vi "main2.vi"() -> ()   [LabVIEW 2016]
uses:
  <vilib>/platform/TimedLoop/XDataNode/XDataNode.xnode
  <vilib>/Platform/TimedLoop/XDataNode/nitl_modes.ctl
  <vilib>/Platform/TimedLoop/XDataNode/XDNodeRunTimeDep.lvlib
  <vilib>/Platform/TimedLoop/XDataNode/wakeup.ctl
  <vilib>/Platform/TimedLoop/XDataNode/timing_clust.ctl
panel:
  in  "retake readings":bool
  in  "Multimeter\nMeasurement":u16(ring) caption="Measurement" items=["DC Voltage (50 A - 50 mV Shunt)", "DC Current (3 A Terminal)", "DC Current (10 A Terminal)", "AC Voltage (50 A - 50 mV Shunt)", "AC Current (3 A Terminal)", "AC Current (10 A Terminal)", "DC Voltage (other)", "AC Voltage (other)", "Continuity", "Diode", "Frequency", "Resistance 4-wire", "Period", "Resistance 2-wire", "Temperature", "DC Voltage Ratio", "Capacitance"]
  in  "zero Hall sensor 3":bool
  in  "zero Hall sensor 2":bool
  in  "zero Hall sensor 1":bool
  in  "start measurement":bool
  in  "initalize instuments":bool
  in  "take readings":bool
  in  "stop":bool
  in  "duration":dbl format="%<%H:%M:%S>t"
  in  "number of readings":i32
  in  "temperature monitor.on":bool
  in  "multimeter.on":bool
  in  "gaussmeter 3.on":bool
  in  "gaussmeter 2.on":bool
  in  "gaussmeter 1.on":bool
  out "status temperature monitor":bool
  out "status multimeter":bool
  out "status gaussmeter 3":bool
  out "status gaussmeter 2":bool
  out "status gaussmeter 1":bool
  in  "VISA resource name temperature monitor":refnum<visa-resource-name>
  in  "VISA resource name multimeter":refnum<visa-resource-name>
  in  "VISA resource name gaussmeter 3":refnum<visa-resource-name>
  in  "VISA resource name gaussmeter 2":refnum<visa-resource-name>
  in  "VISA resource name gaussmeter 1":refnum<visa-resource-name>
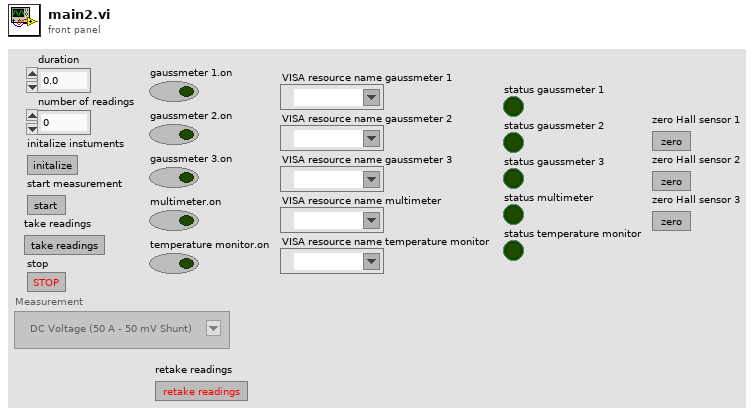
[diagram p1: front panel]
types:
  T1 = enum8{"Enabled", "Disabled", "Disabled and Grayed Out"}
  T2 = typedef "XDNodeRunTimeDep.lvlib/timing_clust.ctl" = cluster{"Expected End [f-1]":u64, "Actual End [f-1]":u64, "Finished Late? [f-1]":bool, "Expected End [i-1]":u64, "Actual End [i-1]":u64, "Finished Late? [i-1]":bool, "Expected Start [i]":u64, "Actual Start [i]":u64, "Expected Start [f]":u64, "Actual Start [f]":u64, "Source Name":string, "Structure Name":string, "Period":i64, "Deadline":i64, "Offset":i64, "Start":i64, "Priority":i32, "Timeout":i32, "Mode":T3, "Wakeup Reason":T4, "Error":errorcluster, "Source Type":string, "Secondary Source Type":string, "Global End Time":u64, "Global Start Time":u64, "Frame Duration":u64, "Iteration Duration":u64, "Assigned CPU":i32, "I/O Scan Engine Mode":u32}
  T3 = typedef "XDNodeRunTimeDep.lvlib/nitl_modes.ctl" = enum32{"No Change", "Process missed periods, maintain original phase", "Discard missed periods, maintain original phase", "Process missed periods, ignore original phase", "Discard missed periods, ignore original phase"}
  T4 = typedef "XDNodeRunTimeDep.lvlib/wakeup.ctl" = enum32{"Normal", "Aborted", "Asynchronous wakeup", "Timing source error", "Timed loop error", "Timeout"}
  T5 = cluster{"gaussmeter 1":cluster{"VISA recourse name":refnum<visa-resource-name>, "on":bool, "header text":string, "units":i32, "initalization successfull":bool}, "gaussmeter 2":cluster{"VISA recourse name":refnum<visa-resource-name>, "on":bool, "header text":string, "units":i32, "initalization successfull":bool}, "gaussmeter 3":cluster{"VISA recourse name":refnum<visa-resource-name>, "on":bool, "header text":string, "units":i32, "initalization successfull":bool}, "multimeter":cluster{"VISA recourse name":refnum<visa-resource-name>, "on":bool, "header text":string, "units":i32, "initalization successfull":bool}, "temperature monitor":cluster{"VISA recourse name":refnum<visa-resource-name>, "on":bool, "header text":string, "units":i32, "initalization successfull":bool}, "duration":cluster{"not zero":bool, "duration":dbl, "start time":dbl}}
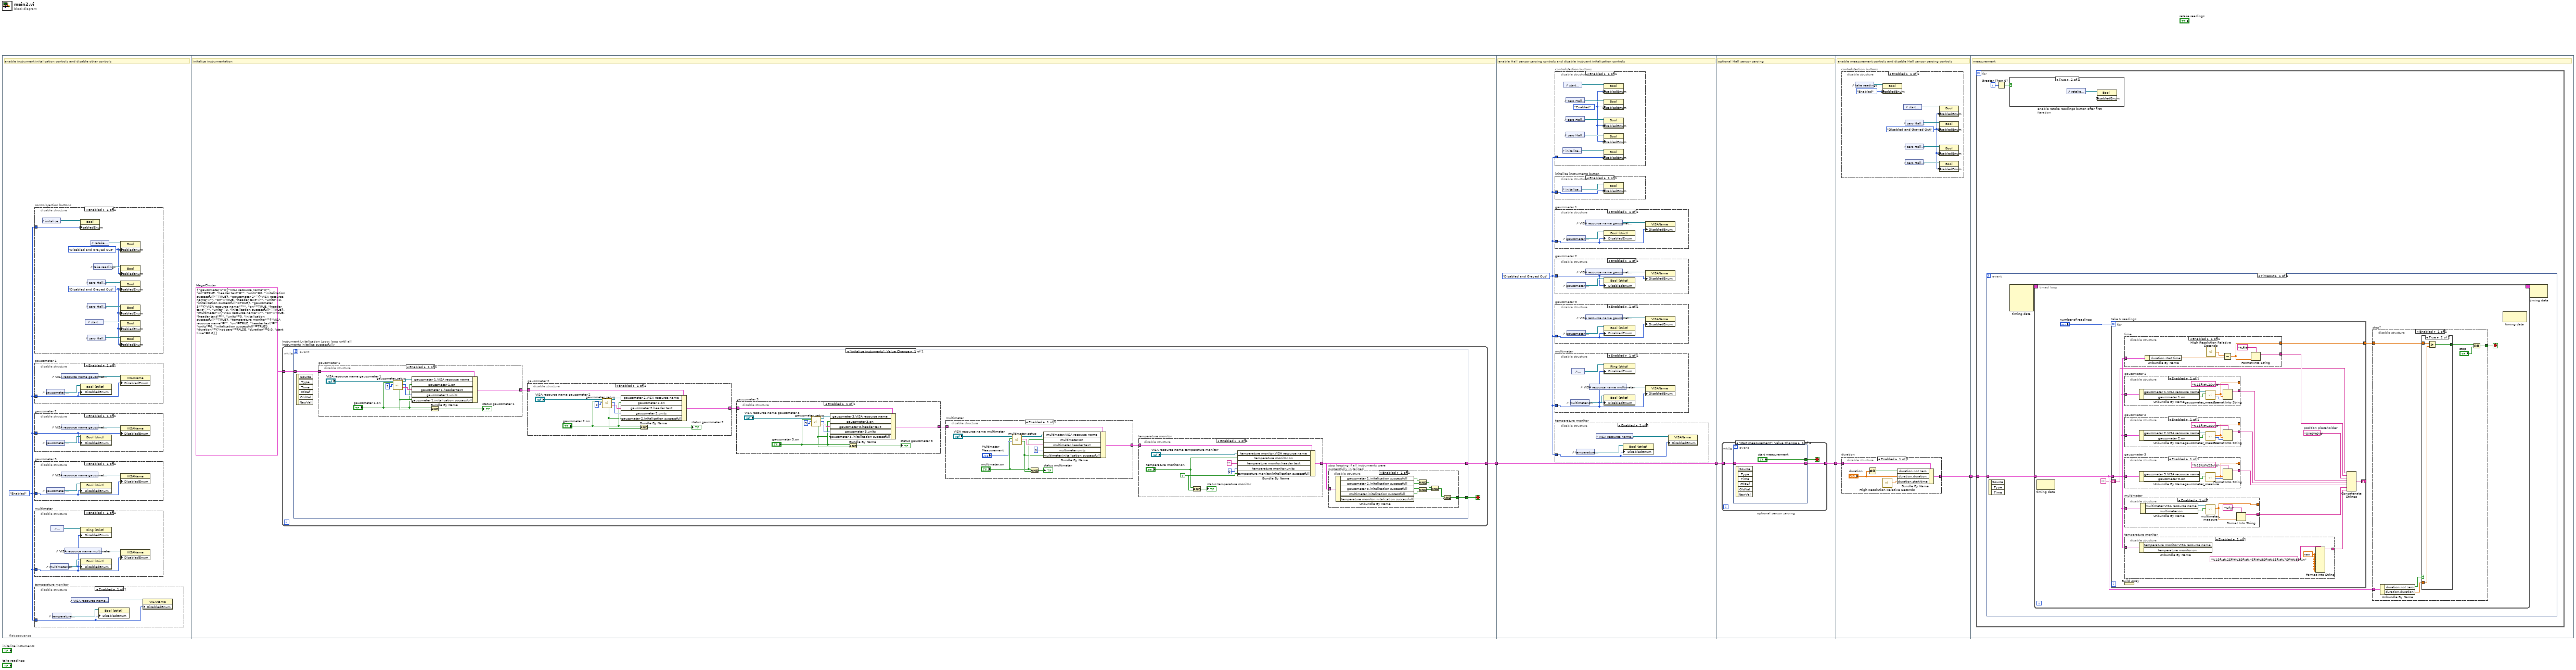
[diagram p0: block diagram]
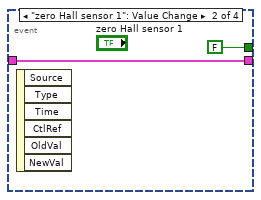
[diagram p2: hidden frame]
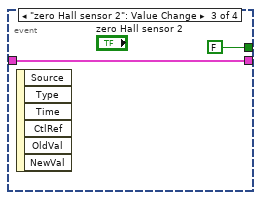
[diagram p3: hidden frame]
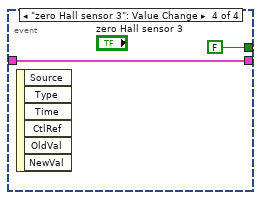
[diagram p4: hidden frame]
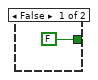
[diagram p6: hidden frame]
diagram:
  n1 = flat-sequence {
    tunnel: [w33] -> w2
    tunnel: w2 -> [w103]
    tunnel: [w103] -> w1
    tunnel: [w130] -> w3
    tunnel: w1 -> [w129]
    tunnel: [w143] -> w4
    tunnel: w3 -> [w142]
    tunnel: w4 -> [w156]
    frame #0 {
      w5 = T1."Enabled" ("Disabled")
      # "enable instrument initalization controls and disable other controls"
      n2 = disable-structure "controls/action buttons" shown="Enabled" {
        disable-tunnel: w5 -> [w12]
        frame Enabled {
          w6 = T1."Disabled and Grayed Out" ("Disabled")
          w8 = T1."Disabled and Grayed Out" ("Disabled")
          n3 = control-ref of="initalize instuments"() -> (w13:refnum<vi>)
          n4 = property class="Bool"(reference=w13, "DisabledEnum"=w12) -> ()  [unwired: 1 in, 2 out]
          n5 = control-ref of="start measurement"() -> (w15:refnum<vi>)
          n6 = control-ref of="zero Hall sensor 2"() -> (w10:refnum<vi>)
          n7 = control-ref of="zero Hall sensor 1"() -> (w11:refnum<vi>)
          n8 = control-ref of="zero Hall sensor 3"() -> (w9:refnum<vi>)
          n9 = control-ref of="retake readings"() -> (w7:refnum<vi>)
          n10 = control-ref of="take readings"() -> (w14:refnum<vi>)
          n11 = property class="Bool"(reference=w7, "DisabledEnum"=w6) -> ()  [unwired: 1 in, 2 out]
          n12 = property class="Bool"(reference=w14, "DisabledEnum"=w6) -> ()  [unwired: 1 in, 2 out]
          n13 = property class="Bool"(reference=w10, "DisabledEnum"=w8) -> ()  [unwired: 1 in, 2 out]
          n14 = property class="Bool"(reference=w11, "DisabledEnum"=w8) -> ()  [unwired: 1 in, 2 out]
          n15 = property class="Bool"(reference=w15, "DisabledEnum"=w8) -> ()  [unwired: 1 in, 2 out]
          n16 = property class="Bool"(reference=w9, "DisabledEnum"=w8) -> ()  [unwired: 1 in, 2 out]
        }
      }
      n17 = disable-structure "gaussmeter 1" shown="Enabled" {
        disable-tunnel: w5 -> [w29]
        frame Enabled {
          n18 = control-ref of="gaussmeter 1.on"() -> (w30:refnum<vi>)
          n19 = control-ref of="VISA resource name gaussmeter 1"() -> (w31:refnum<vi>)
          n20 = property class="Bool (strict)"(reference=w30, "DisabledEnum"=w29) -> ()  [unwired: 1 in, 2 out]
          n21 = property class="VISAName"(reference=w31, "DisabledEnum"=w29) -> ()  [unwired: 1 in, 2 out]
        }
      }
      n22 = disable-structure "gaussmeter 2" shown="Enabled" {
        disable-tunnel: w5 -> [w26]
        frame Enabled {
          n23 = control-ref of="gaussmeter 2.on"() -> (w27:refnum<vi>)
          n24 = control-ref of="VISA resource name gaussmeter 2"() -> (w28:refnum<vi>)
          n25 = property class="Bool (strict)"(reference=w27, "DisabledEnum"=w26) -> ()  [unwired: 1 in, 2 out]
          n26 = property class="VISAName"(reference=w28, "DisabledEnum"=w26) -> ()  [unwired: 1 in, 2 out]
        }
      }
      n27 = disable-structure "gaussmeter 3" shown="Enabled" {
        disable-tunnel: w5 -> [w16]
        frame Enabled {
          n28 = control-ref of="gaussmeter 3.on"() -> (w17:refnum<vi>)
          n29 = control-ref of="VISA resource name gaussmeter 3"() -> (w18:refnum<vi>)
          n30 = property class="Bool (strict)"(reference=w17, "DisabledEnum"=w16) -> ()  [unwired: 1 in, 2 out]
          n31 = property class="VISAName"(reference=w18, "DisabledEnum"=w16) -> ()  [unwired: 1 in, 2 out]
        }
      }
      n32 = disable-structure "multimeter" shown="Enabled" {
        disable-tunnel: w5 -> [w22]
        frame Enabled {
          n33 = control-ref of="multimeter.on"() -> (w24:refnum<vi>)
          n34 = control-ref of="Multimeter\nMeasurement"() -> (w25:refnum<vi>)
          n35 = control-ref of="VISA resource name multimeter"() -> (w23:refnum<vi>)
          n36 = property class="Ring (strict)"(reference=w25, "DisabledEnum"=w22) -> ()  [unwired: 1 in, 2 out]
          n37 = property class="Bool (strict)"(reference=w24, "DisabledEnum"=w22) -> ()  [unwired: 1 in, 2 out]
          n38 = property class="VISAName"(reference=w23, "DisabledEnum"=w22) -> ()  [unwired: 1 in, 2 out]
        }
      }
      n39 = disable-structure "temperature monitor" shown="Enabled" {
        disable-tunnel: w5 -> [w21]
        frame Enabled {
          n40 = control-ref of="temperature monitor.on"() -> (w19:refnum<vi>)
          n41 = control-ref of="VISA resource name temperature monitor"() -> (w20:refnum<vi>)
          n42 = property class="Bool (strict)"(reference=w19, "DisabledEnum"=w21) -> ()  [unwired: 1 in, 2 out]
          n43 = property class="VISAName"(reference=w20, "DisabledEnum"=w21) -> ()  [unwired: 1 in, 2 out]
        }
      }
    }
    frame #1 {
      w32 = T5 {"gaussmeter 1"={"VISA recourse name"="", "on"=TRUE, "header text"="", "units"=0, "initalization successfull"=TRUE}, "gaussmeter 2"={"VISA recourse name"="", "on"=TRUE, "header text"="", "units"=0, "initalization successfull"=TRUE}, "gaussmeter 3"={"VISA recourse name"="", "on"=TRUE, "header text"="", "units"=0, "initalization successfull"=TRUE}, "multimeter"={"VISA recourse name"="", "on"=TRUE, "header text"="", "units"=0, "initalization successfull"=TRUE}, "temperature monitor"={"VISA recourse name"="", "on"=TRUE, "header text"="", "units"=0, "initalization successfull"=TRUE}, "duration"={"not zero"=FALSE, "duration"=0.0, "start time"=0.0}}  # MegaCluster
      # "initalize instrumentation"
      n44 = while "Instrument Lnitalization Loop: loop until all instruments initalize successfully" {
        tunnel: [w35] -> w33
        tunnel: w32 -> [w36]
        stop <- w34 stop-if-true
        n45 = event shown="[0] \"initalize instuments\": Value Change" {
          selector: _ -> [_]
          dyn-events: _ -> [_]
          timeout: _ -> [_]
          tunnel: w36 -> [w39]
          tunnel: [w38] -> w35
          tunnel: [w37] -> w34
          event "initalize instuments": Value Change {
            n46 = event-data() -> ()  [unwired: 1 in, 6 out]
            n47 = disable-structure "gaussmeter 1" shown="Enabled" {
              disable-tunnel: [w81] -> w43
              disable-tunnel: w39 -> [w80]
              frame Enabled {
                n48 = call "gaussmeter_setup.vi"("VISA resource name Gaussmeter"="VISA resource name gaussmeter 1", "Switch Gaussmeter"="gaussmeter 1.on", "Gaussmeter Number"=u8 1) -> ("Status Gaussmeter"=w73:bool, "Gaussmeter VISA resource name out"=w77:refnum<visa-resource-name>, "Field Units"=w75:u16, "Text Output"=w76:string)  [unwired: 6 in, 7 out]
                n49 = Bundle By Name(cluster=w80, "gaussmeter 1.VISA recourse name"=w77, "gaussmeter 1.on"="gaussmeter 1.on", "gaussmeter 1.header text"=w76, "gaussmeter 1.units"=w75, "gaussmeter 1.initalization successfull"=w73) -> (w81:T5)
                n50 = And(x="gaussmeter 1.on", y=w73) -> (x .and. y?=→"status gaussmeter 1":bool)
              }
            }
            n51 = disable-structure "gaussmeter 2" shown="Enabled" {
              disable-tunnel: [w100] -> w42
              disable-tunnel: w43 -> [w101]
              frame Enabled {
                n52 = call "gaussmeter_setup.vi"("VISA resource name Gaussmeter"="VISA resource name gaussmeter 2", "Switch Gaussmeter"="gaussmeter 2.on", "Gaussmeter Number"=u8 2) -> ("Status Gaussmeter"=w93:bool, "Gaussmeter VISA resource name out"=w97:refnum<visa-resource-name>, "Field Units"=w96:u16, "Text Output"=w95:string)  [unwired: 6 in, 7 out]
                n53 = Bundle By Name(cluster=w101, "gaussmeter 2.VISA recourse name"=w97, "gaussmeter 2.on"="gaussmeter 2.on", "gaussmeter 2.header text"=w95, "gaussmeter 2.units"=w96, "gaussmeter 2.initalization successfull"=w93) -> (w100:T5)
                n54 = And(x="gaussmeter 2.on", y=w93) -> (x .and. y?=→"status gaussmeter 2":bool)
              }
            }
            n55 = disable-structure "gaussmeter 3" shown="Enabled" {
              disable-tunnel: [w91] -> w41
              disable-tunnel: w42 -> [w90]
              frame Enabled {
                n56 = call "gaussmeter_setup.vi"("VISA resource name Gaussmeter"="VISA resource name gaussmeter 3", "Switch Gaussmeter"="gaussmeter 3.on", "Gaussmeter Number"=u8 3) -> ("Status Gaussmeter"=w82:bool, "Gaussmeter VISA resource name out"=w88:refnum<visa-resource-name>, "Field Units"=w85:u16, "Text Output"=w86:string)  [unwired: 6 in, 7 out]
                n57 = Bundle By Name(cluster=w90, "gaussmeter 3.VISA recourse name"=w88, "gaussmeter 3.on"="gaussmeter 3.on", "gaussmeter 3.header text"=w86, "gaussmeter 3.units"=w85, "gaussmeter 3.initalization successfull"=w82) -> (w91:T5)
                n58 = And(x="gaussmeter 3.on", y=w82) -> (x .and. y?=→"status gaussmeter 3":bool)
              }
            }
            n59 = disable-structure "multimeter" shown="Enabled" {
              disable-tunnel: [w71] -> w40
              disable-tunnel: w41 -> [w70]
              frame Enabled {
                n60 = call "multimeter_setup.vi"("Measurement"="Multimeter\nMeasurement", "Switch"="multimeter.on", "VISA resource name"="VISA resource name multimeter") -> ("status"=w62:bool, "text"=w66:string, "VISA resource name out"=w67:refnum<visa-resource-name>)  [unwired: 5 in, 1 out]
                n61 = And(x="multimeter.on", y=w62) -> (x .and. y?=→"status multimeter":bool)
                n62 = Bundle By Name(cluster=w70, "multimeter.VISA recourse name"=w67, "multimeter.on"="multimeter.on", "multimeter.header text"=w66, "multimeter.units"=0, "multimeter.initalization successfull"=w62) -> (w71:T5)
              }
            }
            n63 = disable-structure "temperature monitor" shown="Enabled" {
              disable-tunnel: [w61] -> w38
              disable-tunnel: w40 -> [w60]
              frame Enabled {
                w55 = TRUE
                n64 = And(x="temperature monitor.on", y=w55) -> (x .and. y?=→"status temperature monitor":bool)
                n65 = Bundle By Name(cluster=w60, "temperature monitor.VISA recourse name"="VISA resource name temperature monitor", "temperature monitor.on"="temperature monitor.on", "temperature monitor.header text"="", "temperature monitor.units"=0, "temperature monitor.initalization successfull"=w55) -> (w61:T5)
              }
            }
            n66 = disable-structure "stop looping if all instruments were successfully initalized" shown="Enabled" {
              disable-tunnel: w38 -> [w50]
              disable-tunnel: [w44] -> w37
              frame Enabled {
                n67 = Unbundle By Name(w50) -> ("gaussmeter 1.initalization successfull"=w49:bool, "gaussmeter 2.initalization successfull"=w48:bool, "gaussmeter 3.initalization successfull"=w47:bool, "multimeter.initalization successfull"=w46:bool, "temperature monitor.initalization successfull"=w45:bool)
                n68 = And(x=w49, y=w48) -> (x .and. y?=w52:bool)
                n69 = And(x=w47, y=w46) -> (x .and. y?=w51:bool)
                n70 = And(x=w52, y=w51) -> (x .and. y?=w53:bool)
                n71 = And(x=w53, y=w45) -> (x .and. y?=w44:bool)
              }
            }
          }
        }
      }
    }
    frame #2 {
      w102 = T1."Disabled and Grayed Out" ("Disabled")
      # "enable Hall sensor zeroing controls and disable instruent initalization controls"
      n72 = disable-structure "controls/action buttons" shown="Enabled" {
        disable-tunnel: w102 -> [w108]
        frame Enabled {
          w104 = T1."Enabled" ("Disabled")
          n73 = control-ref of="initalize instuments"() -> (w109:refnum<vi>)
          n74 = control-ref of="start measurement"() -> (w110:refnum<vi>)
          n75 = control-ref of="zero Hall sensor 2"() -> (w106:refnum<vi>)
          n76 = control-ref of="zero Hall sensor 1"() -> (w107:refnum<vi>)
          n77 = control-ref of="zero Hall sensor 3"() -> (w105:refnum<vi>)
          n78 = property class="Bool"(reference=w110, "DisabledEnum"=w104) -> ()  [unwired: 1 in, 2 out]
          n79 = property class="Bool"(reference=w106, "DisabledEnum"=w104) -> ()  [unwired: 1 in, 2 out]
          n80 = property class="Bool"(reference=w107, "DisabledEnum"=w104) -> ()  [unwired: 1 in, 2 out]
          n81 = property class="Bool"(reference=w105, "DisabledEnum"=w104) -> ()  [unwired: 1 in, 2 out]
          n82 = property class="Bool"(reference=w109, "DisabledEnum"=w108) -> ()  [unwired: 1 in, 2 out]
        }
      }
      n83 = disable-structure "initalize instruments button" shown="Enabled" {
        disable-tunnel: w102 -> [w112]
        frame Enabled {
          n84 = control-ref of="initalize instuments"() -> (w111:refnum<vi>)
          n85 = property class="Bool"(reference=w111, "DisabledEnum"=w112) -> ()  [unwired: 1 in, 2 out]
        }
      }
      n86 = disable-structure "gaussmeter 1" shown="Enabled" {
        disable-tunnel: w102 -> [w126]
        frame Enabled {
          n87 = control-ref of="gaussmeter 1.on"() -> (w127:refnum<vi>)
          n88 = control-ref of="VISA resource name gaussmeter 1"() -> (w128:refnum<vi>)
          n89 = property class="Bool (strict)"(reference=w127, "DisabledEnum"=w126) -> ()  [unwired: 1 in, 2 out]
          n90 = property class="VISAName"(reference=w128, "DisabledEnum"=w126) -> ()  [unwired: 1 in, 2 out]
        }
      }
      n91 = disable-structure "gaussmeter 2" shown="Enabled" {
        disable-tunnel: w102 -> [w123]
        frame Enabled {
          n92 = control-ref of="gaussmeter 2.on"() -> (w124:refnum<vi>)
          n93 = control-ref of="VISA resource name gaussmeter 2"() -> (w125:refnum<vi>)
          n94 = property class="Bool (strict)"(reference=w124, "DisabledEnum"=w123) -> ()  [unwired: 1 in, 2 out]
          n95 = property class="VISAName"(reference=w125, "DisabledEnum"=w123) -> ()  [unwired: 1 in, 2 out]
        }
      }
      n96 = disable-structure "gaussmeter 3" shown="Enabled" {
        disable-tunnel: w102 -> [w113]
        frame Enabled {
          n97 = control-ref of="gaussmeter 3.on"() -> (w114:refnum<vi>)
          n98 = control-ref of="VISA resource name gaussmeter 3"() -> (w115:refnum<vi>)
          n99 = property class="Bool (strict)"(reference=w114, "DisabledEnum"=w113) -> ()  [unwired: 1 in, 2 out]
          n100 = property class="VISAName"(reference=w115, "DisabledEnum"=w113) -> ()  [unwired: 1 in, 2 out]
        }
      }
      n101 = disable-structure "multimeter" shown="Enabled" {
        disable-tunnel: w102 -> [w119]
        frame Enabled {
          n102 = control-ref of="multimeter.on"() -> (w121:refnum<vi>)
          n103 = control-ref of="Multimeter\nMeasurement"() -> (w122:refnum<vi>)
          n104 = control-ref of="VISA resource name multimeter"() -> (w120:refnum<vi>)
          n105 = property class="Ring (strict)"(reference=w122, "DisabledEnum"=w119) -> ()  [unwired: 1 in, 2 out]
          n106 = property class="Bool (strict)"(reference=w121, "DisabledEnum"=w119) -> ()  [unwired: 1 in, 2 out]
          n107 = property class="VISAName"(reference=w120, "DisabledEnum"=w119) -> ()  [unwired: 1 in, 2 out]
        }
      }
      n108 = disable-structure "temperature monitor" shown="Enabled" {
        disable-tunnel: w102 -> [w118]
        frame Enabled {
          n109 = control-ref of="temperature monitor.on"() -> (w116:refnum<vi>)
          n110 = control-ref of="VISA resource name temperature monitor"() -> (w117:refnum<vi>)
          n111 = property class="Bool (strict)"(reference=w116, "DisabledEnum"=w118) -> ()  [unwired: 1 in, 2 out]
          n112 = property class="VISAName"(reference=w117, "DisabledEnum"=w118) -> ()  [unwired: 1 in, 2 out]
        }
      }
    }
    frame #3 {
      # "optional Hall sensor zeroing"
      n113 = while "optional sensor zeroing" {
        tunnel: [w132] -> w130
        tunnel: w129 -> [w133]
        stop <- w131 stop-if-true
        n114 = event shown="[0] \"start measurement\": Value Change" {
          selector: _ -> [_ _ _ _]
          dyn-events: _ -> [_ _ _ _]
          timeout: _ -> [_ _ _ _]
          tunnel: w133 -> [w134 w137 w139 w141]
          tunnel: [w134 w137 w139 w141] -> w132
          tunnel: ["start measurement" FALSE ("start measurement") FALSE ("start measurement") FALSE ("start measurement")] -> w131
          event "start measurement": Value Change {
            n115 = event-data() -> ()  [unwired: 1 in, 6 out]
          }
          event "zero Hall sensor 1": Value Change {
            n116 = event-data() -> ()  [unwired: 1 in, 6 out]
          }
          event "zero Hall sensor 2": Value Change {
            n117 = event-data() -> ()  [unwired: 1 in, 6 out]
          }
          event "zero Hall sensor 3": Value Change {
            n118 = event-data() -> ()  [unwired: 1 in, 6 out]
          }
        }
      }
    }
    frame #4 {
      # "enable measurement controls and disable Hall sensor zeroing controls"
      n119 = disable-structure "controls/action buttons" shown="Enabled" {
        frame Enabled {
          w145 = T1."Disabled and Grayed Out" ("Disabled")
          n120 = control-ref of="take readings"() -> (w149:refnum<vi>)
          n121 = property class="Bool"(reference=w149, "DisabledEnum"=T1."Enabled" ("Disabled")) -> ()  [unwired: 1 in, 2 out]
          n122 = control-ref of="start measurement"() -> (w150:refnum<vi>)
          n123 = control-ref of="zero Hall sensor 2"() -> (w147:refnum<vi>)
          n124 = control-ref of="zero Hall sensor 1"() -> (w148:refnum<vi>)
          n125 = control-ref of="zero Hall sensor 3"() -> (w146:refnum<vi>)
          n126 = property class="Bool"(reference=w150, "DisabledEnum"=w145) -> ()  [unwired: 1 in, 2 out]
          n127 = property class="Bool"(reference=w147, "DisabledEnum"=w145) -> ()  [unwired: 1 in, 2 out]
          n128 = property class="Bool"(reference=w148, "DisabledEnum"=w145) -> ()  [unwired: 1 in, 2 out]
          n129 = property class="Bool"(reference=w146, "DisabledEnum"=w145) -> ()  [unwired: 1 in, 2 out]
        }
      }
      n130 = disable-structure "duration" shown="Enabled" {
        disable-tunnel: [w155] -> w143
        disable-tunnel: w142 -> [w151]
        frame Enabled {
          n131 = Not Equal To 0?(x="duration") -> (x != 0?=w154:bool)
          n132 = call <vilib>:"High Resolution Relative Seconds.vi"() -> ("relative seconds"=w152:dbl)
          n133 = Bundle By Name(cluster=w151, "duration.not zero"=w154, "duration.duration"="duration", "duration.start time"=w152) -> (w155:T5)
        }
      }
    }
    frame #5 {
      # "measurement"
      n134 = for {
        tunnel: w156 -> [w159]
        i -> [w157]
        n135 = event shown="[0] Timeout" {
          selector: _ -> [_]
          dyn-events: _ -> [_]
          timeout: _ -> [_]
          tunnel: w159 -> [w161]
          event Timeout {
            n136 = event-data() -> ()  [unwired: 1 in, 3 out]
            n137 = node-c288() -> (w163:T2)  [unwired: 4 in]
            n138 = timed-loop {
              timing: w163 -> [_]
              timing-out: [_] -> w162
              tunnel: w161 -> [w166]
              stop <- w167 stop-if-true
              n139 = node-c288() -> ()  [unwired: 1 in, 1 out]
              n140 = for "take N readings" {
                N: "number of readings" -> [_]
                tunnel: w166 -> [w190]
                shift-right: [w181] -> _
                shift-left: "" -> [w182]
                tunnel: [w180] -> w164
                w188 = "0\\t0\\t0\\t"  # position placeholder
                n141 = disable-structure "time" shown="Enabled" {
                  disable-tunnel: [w223] -> w180
                  disable-tunnel: w190 -> [w225]
                  disable-tunnel: [w222] -> w189
                  frame Enabled {
                    n142 = Unbundle By Name(w225) -> ("duration.start time"=w226:dbl)
                    n143 = call <vilib>:"High Resolution Relative Seconds.vi"() -> ("relative seconds"=w227:dbl)
                    n144 = Subtract(x=w227, y=w226) -> (x-y=w223:dbl)
                    n145 = Format Into String(format string="%f\\t", w223) -> (resulting string=w222:string)  [unwired: 2 in, 1 out]
                  }
                }
                n146 = disable-structure "gaussmeter 1" shown="Enabled" {
                  disable-tunnel: w190 -> [w221]
                  disable-tunnel: [w216] -> w187
                  disable-tunnel: [w215] -> _
                  frame Enabled {
                    n147 = Unbundle By Name(w221) -> ("gaussmeter 1.VISA recourse name"=w220:refnum<visa-resource-name>, "gaussmeter 1.on"=w219:bool)
                    n148 = call "gaussmeter_measure.vi"("Switch Gaussmeter"=w219, "VISA resource name"=w220) -> ("Field Range"=w217:u16, "Field Reading"=w215:dbl)  [unwired: 5 in, 3 out]
                    n149 = Format Into String(format string="%1$f\\t%2$u\\t", w215, w217) -> (resulting string=w216:string)  [unwired: 2 in, 1 out]
                  }
                }
                n150 = disable-structure "gaussmeter 2" shown="Enabled" {
                  disable-tunnel: w190 -> [w214]
                  disable-tunnel: [w209] -> w186
                  disable-tunnel: [w208] -> _
                  frame Enabled {
                    n151 = Unbundle By Name(w214) -> ("gaussmeter 2.VISA recourse name"=w213:refnum<visa-resource-name>, "gaussmeter 2.on"=w212:bool)
                    n152 = call "gaussmeter_measure.vi"("Switch Gaussmeter"=w212, "VISA resource name"=w213) -> ("Field Range"=w210:u16, "Field Reading"=w208:dbl)  [unwired: 5 in, 3 out]
                    n153 = Format Into String(format string="%1$f\\t%2$u\\t", w208, w210) -> (resulting string=w209:string)  [unwired: 2 in, 1 out]
                  }
                }
                n154 = disable-structure "gaussmeter 3" shown="Enabled" {
                  disable-tunnel: w190 -> [w207]
                  disable-tunnel: [w202] -> w185
                  disable-tunnel: [w201] -> _
                  frame Enabled {
                    n155 = Unbundle By Name(w207) -> ("gaussmeter 3.VISA recourse name"=w206:refnum<visa-resource-name>, "gaussmeter 3.on"=w205:bool)
                    n156 = call "gaussmeter_measure.vi"("Switch Gaussmeter"=w205, "VISA resource name"=w206) -> ("Field Range"=w203:u16, "Field Reading"=w201:dbl)  [unwired: 5 in, 3 out]
                    n157 = Format Into String(format string="%1$f\\t%2$u\\t", w201, w203) -> (resulting string=w202:string)  [unwired: 2 in, 1 out]
                  }
                }
                n158 = disable-structure "multimeter" shown="Enabled" {
                  disable-tunnel: w190 -> [w200]
                  disable-tunnel: [w196] -> w184
                  disable-tunnel: [w195] -> _
                  frame Enabled {
                    n159 = Unbundle By Name(w200) -> ("multimeter.VISA recourse name"=w199:refnum<visa-resource-name>, "multimeter.on"=w198:bool)
                    n160 = call "multimeter_measure.vi"("Switch Multimeter"=w198, "VISA resource name"=w199) -> ("Reading"=w195:dbl)  [unwired: 6 in, 3 out]
                    n161 = Format Into String(format string="%f\\t", w195) -> (resulting string=w196:string)  [unwired: 2 in, 1 out]
                  }
                }
                n162 = disable-structure "temperature monitor" shown="Enabled" {
                  disable-tunnel: w190 -> [w194]
                  disable-tunnel: [w192] -> w183
                  frame Enabled {
                    w191 = nan
                    n163 = Unbundle By Name(w194) -> ()  [unwired: 2 out]
                    n164 = Format Into String(format string="%1$f\\t%2$f\\t%3$f\\t%4$f\\t%5$f\\t%6$f\\t%7$f\\t%8$f\\n", w191, w191, w191, w191, w191, w191, w191, w191) -> (resulting string=w192:string)  [unwired: 2 in, 1 out]
                  }
                }
                n165 = Build Array() -> ()  [unwired: 1 in, 1 out]
                n166 = Concatenate Strings(w182, w189, w188, w187, w186, w185, w184, w183) -> (w181:string)
              }
              n167 = disable-structure "stop?" shown="Enabled" {
                disable-tunnel: [w175] -> w167
                disable-tunnel: w166 -> [w172]
                disable-tunnel: w164 -> [w169]
                frame Enabled {
                  n168 = Unbundle By Name(w172) -> ("duration.not zero"=w173:bool, "duration.duration"=w170:dbl)
                  n169 = case shown="True" w173 {
                    tunnel: [FALSE w179] -> w174
                    tunnel: w170 -> [_ w178]
                    tunnel: w169 -> [_ w177]
                    frame False {
                    }
                    frame True {
                      n170 = Greater Or Equal?(x=w177, y=w178) -> (x >= y?=w179:bool)
                    }
                  }
                  n171 = Or(x=w174, y="stop") -> (x .or. y?=w175:bool)
                }
              }
              n172 = node-c288() -> ()  [unwired: 1 in, 1 out]
            }
            n173 = node-c288(w162) -> ()  [unwired: 1 out]
          }
        }
        n174 = Greater Than 0?(x=w157) -> (x > 0?=w158:bool)
        n175 = case "enable retake readings button after first iteration" shown="True" w158 {
          frame False {
          }
          frame True {
            n176 = control-ref of="retake readings"() -> (w160:refnum<vi>)
            n177 = property class="Bool" props=["DisabledEnum"](reference=w160) -> ()  [unwired: 2 in, 2 out]
          }
        }
      }
    }
  }
